vi "Atto DRY Interface start Logging.vi"(8 "error in (no error)":errorcluster, 9 "Append":i32, 10 "TimeSelection":u16, 11 "Path":string) -> (0 "error out":errorcluster, 2 "function return":i32, 3 "Path out":string)   [LabVIEW 2016, in "attoDRYLib.lvlib"]
doc: "int32_t __cdecl AttoDRY_Interface_startLogging(char Path[], \n Enum TimeSelection, int Append);"
uses:
  <userlib>/attoDRYLib/attoDRYLib.lvlib
  <userlib>/attoDRYLib/attoDRYLib.dll
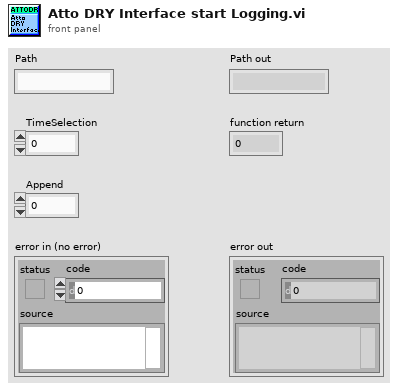
[diagram p1: front panel]
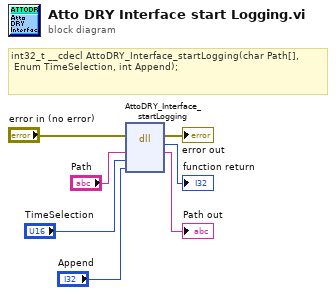
[diagram p0: block diagram]
diagram:
  # "int32_t __cdecl AttoDRY_Interface_startLogging(char Path[], \n\tEnum TimeSelection, int Append);"
  n1 = dll-call lib="C:/Program Files (x86)/National Instruments/LabVIEW 2016/user.lib/attoDRYLib/attoDRYLib.*" fn="AttoDRY_Interface_startLogging"(error in="error in (no error)", "Path"="Path", "TimeSelection"="TimeSelection", "Append"="Append") -> (error out=→"error out":errorcluster, →"function return":i32, "Path"=→"Path out":string)  [unwired: 4 in, 1 out]
